vi "SpaceFlightBookingMarcoGonzalez.vi"() -> ()   [LabVIEW 2012]
panel:
  in  "?":bool
  out "Travel Time (seconds)":i64
  out "Travel Cost (U.S dollars)":i64
  out "Distance from Earth (kilometers)":i64
  in  "Enter Your Weight (kilograms)":dbl
  in  "Select Method of Travel":u16(ring) items=["Saturn V", "Falcon Heavy"]
  in  "Select Destination":u16(ring) items=["Pluto", "Callisto", "Ganymede", "Ceres", "Earth's Moon", "Venus", "Mars", "Titan", "Europa", "Enceladus"]
  # "Click arrow (above) to begin using program.\nHit \"End\" to stop using the program."
  # "Click on scroll \ndown menu to \nsee choices."
  # "Use arrows to \niinput weight or \ntype the number \ninto the box."
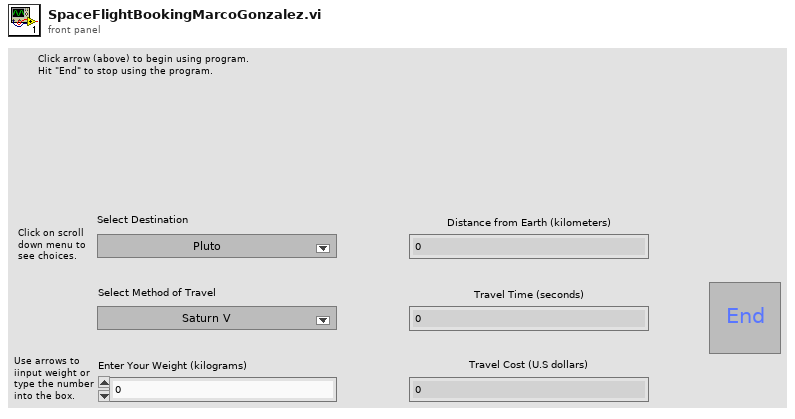
[diagram p1: front panel]
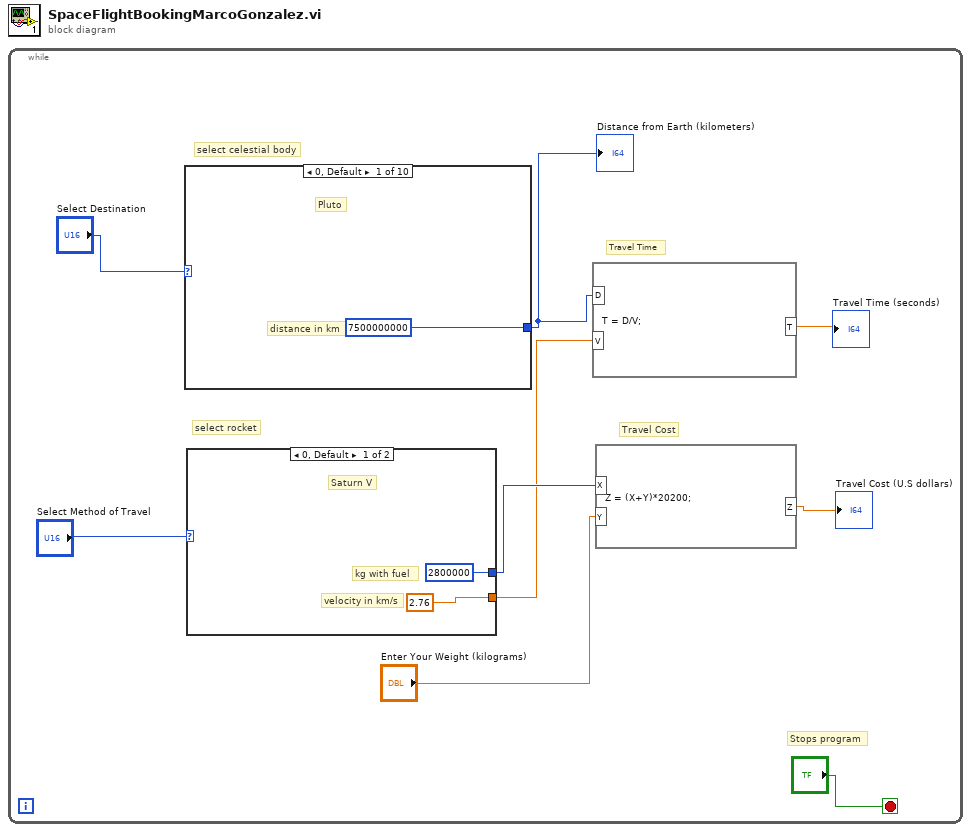
[diagram p0: block diagram]
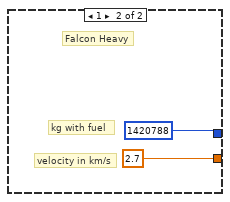
[diagram p2: hidden frame]
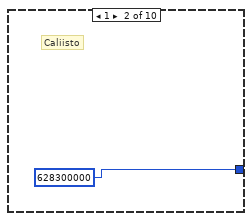
[diagram p3: hidden frame]
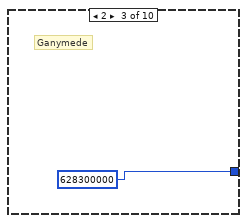
[diagram p4: hidden frame]
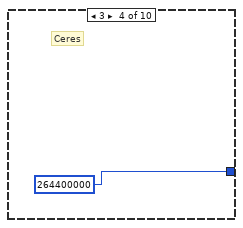
[diagram p5: hidden frame]
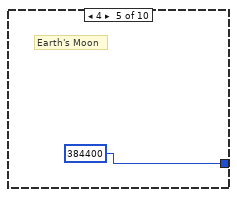
[diagram p6: hidden frame]
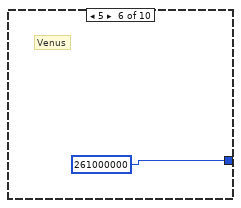
[diagram p7: hidden frame]
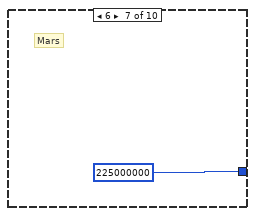
[diagram p8: hidden frame]
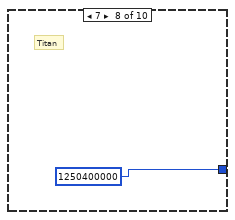
[diagram p9: hidden frame]
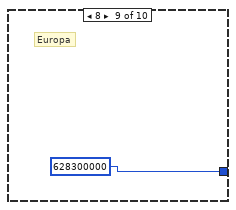
[diagram p10: hidden frame]
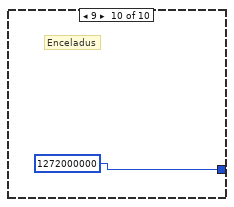
[diagram p11: hidden frame]
diagram:
  n1 = while {
    stop <- "?" stop-if-true
    # "select rocket"
    # "select celestial body"
    # "Stops program"
    # "Travel Cost"
    # "Travel Time"
    n2 = case shown="0, Default" "Select Destination" {
      tunnel: [i64 7500000000 628300000 628300000 264400000 384400 261000000 225000000 1250400000 628300000 1272000000] -> w4
      frame 0, Default {
        # "distance in km"
        # "Pluto"
      }
      frame 1 {
        # "Caliisto"
      }
      frame 2 {
        # "Ganymede"
      }
      frame 3 {
        # "Ceres"
      }
      frame 4 {
        # "Earth's Moon"
      }
      frame 5 {
        # "Venus"
      }
      frame 6 {
        # "Mars"
      }
      frame 7 {
        # "Titan"
      }
      frame 8 {
        # "Europa"
      }
      frame 9 {
        # "Enceladus"
      }
    }
    "Distance from Earth (kilometers)" <- w4
    n3 = case shown="0, Default" "Select Method of Travel" {
      tunnel: [2800000 1420788] -> w7
      tunnel: [2.76 2.7] -> w3
      frame 0, Default {
        # "velocity in km/s"
        # "kg with fuel"
        # "Saturn V"
      }
      frame 1 {
        # "velocity in km/s"
        # "kg with fuel"
        # "Falcon Heavy"
      }
    }
    n4 = formula code="T = D/V;"("V"=w3, "D"=w4) -> ("T"=→"Travel Time (seconds)":dbl)
    n5 = formula code="Z = (X+Y)*20200;"("X"=w7, "Y"="Enter Your Weight (kilograms)") -> ("Z"=→"Travel Cost (U.S dollars)":dbl)
  }
